vi "Get Chnl by Name.vi"(8 "error in (no error)":errorcluster, 10 "Chnl Name":string, 11 "BME_DG_Base in":refnum<class "BME_DG_Base.lvclass">) -> (0 "error out":errorcluster, 1 "found?":bool, 2 "BME_DG_Chnl out":refnum<class "BME_DG_Chnl.lvclass">, 3 "BME_DG_Base out":refnum<class "BME_DG_Base.lvclass">)   [LabVIEW 2009, in "POLARIS BME DG.lvlib" / "BME_DG_Base.lvclass"]
uses:
  BME_DG_Base.lvclass
  BME_DG_Chnl/BME_DG_Chnl.lvclass
  BME_DG_Base.lvclass/BME_DG_Base.ctl
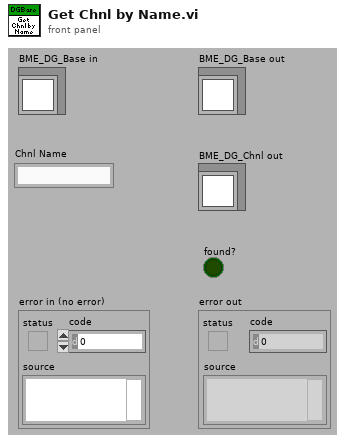
[diagram p1: front panel]
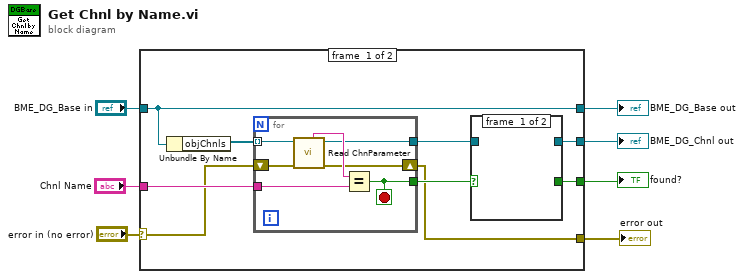
[diagram p0: block diagram]
diagram:
  n1 = case shown="No Error" "error in (no error)" {
    selector: "error in (no error)" -> [w9 w27]
    tunnel: [w8 w27] -> w6
    tunnel: [w16 w26] -> w4
    tunnel: "BME_DG_Base in" -> [w16 w26]
    tunnel: "Chnl Name" -> [w14 _]
    tunnel: [w12 _] -> w2
    tunnel: [w11 _] -> w1
    frame #0 {
      n2 = Unbundle By Name(w16) -> ("objChnls"=w15:refnum<class "BME_DG_Chnl.lvclass">[])
      n3 = for {
        tunnel: w15 -> [w25] mode=indexing
        tunnel: w14 -> [w23]
        tunnel: [w22] -> w13
        tunnel: [w21] -> w10
        shift-right: [w19] -> w8
        shift-left: w9 -> [w20]
        stop <- w22 stop-if-true
        n4 = call-dynamic "Read ChnParameter.vi"("error in (no error)"=w20, "BME_DG_Chnl in"=w25) -> ("error out"=w19:errorcluster, "BME_DG_Chnl out"=w21:refnum<class "BME_DG_Chnl.lvclass">, "Name"=w24:string)  [unwired: 4 in, 3 out]
        n5 = Equal?(x=w24, y=w23) -> (x = y?=w22:bool)
      }
      n6 = case shown="True" w13 {
        selector: w13 -> [_ w18]
        tunnel: [_ w18] -> w12
        tunnel: [_ w17] -> w11
        tunnel: w10 -> [_ w17]
        frame #0 {
        }
        frame #1 {
        }
      }
    }
    frame #1 {
    }
  }
  "error out" <- w6
  "BME_DG_Base out" <- w4
  "found?" <- w2
  "BME_DG_Chnl out" <- w1
